vi "Untitled 2 (SubVI).vi"(0 "16xIQ in":T1[][](array[typedef]), 9 "Array in":bool[](array[boolean])=[FALSE, FALSE, FALSE, FALSE, FALSE, FALSE, FALSE, FALSE, FALSE, FALSE, FALSE, FALSE, FALSE, FALSE, FALSE, FALSE]) -> (8 "Array out":bool[](array[boolean]))   [LabVIEW 2015]
uses:
  DDC_7976R_v1.lvlib
  <instrlib>/_niInstr/DSP/v1/Shared/Public/IQ Data.ctl
  <instrlib>/_niInstr/DSP/v1/Shared/niInstr DSP v1 Shared.lvlib
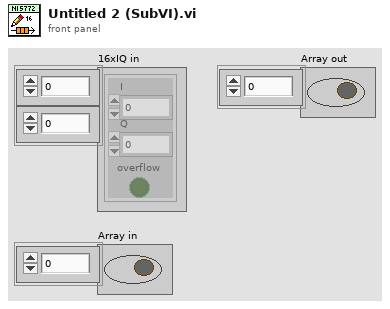
[diagram p1: front panel]
types:
  T1 = typedef "niInstr DSP v1 Shared.lvlib/IQ Data.ctl" = cluster{"I":fxp<+/-,18,1>, "Q":fxp<+/-,18,1>, "overflow":bool}
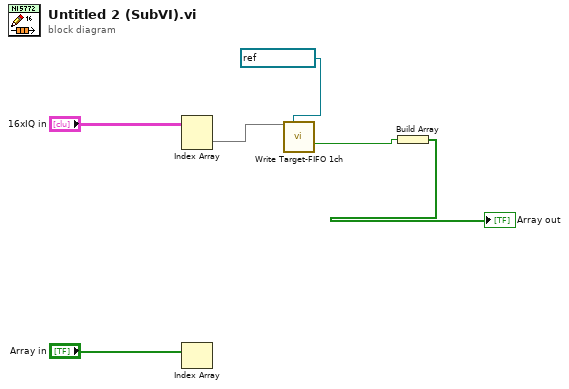
[diagram p0: block diagram]
diagram:
  n1 = Index Array(array="16xIQ in") -> (element=w1:T1[])  [unwired: 2 in]
  n2 = Index Array(array="Array in") -> ()  [unwired: 1 in, 1 out]
  n3 = call "Write Target-FIFO 1ch.vi"(0:w1, "FIFO In"=refnum<k21> "FIFO-000") -> ("Timed Out?"=w5:bool)  [unwired: 13 in]
  n4 = Build Array(w5) -> (→"Array out":bool[])
